vi "MH_WRabbitGetSFPData.vi"(8 "error in (no error)":errorcluster, 11 "devidx":i32) -> (0 "error out":errorcluster, 1 "dRxs":i32[](array[numeric]), 2 "dTxs":i32[](array[numeric]), 3 "return type":i32, 4 "alphas":i32[](array[numeric]), 5 "sfpnames":string[](array[string]))   [LabVIEW 2019]
uses:
  MH_DllPath_global.vi
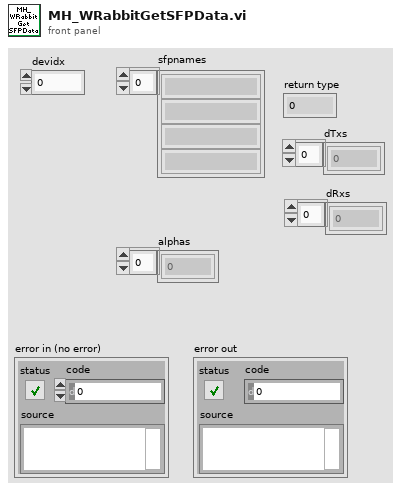
[diagram p1: front panel]
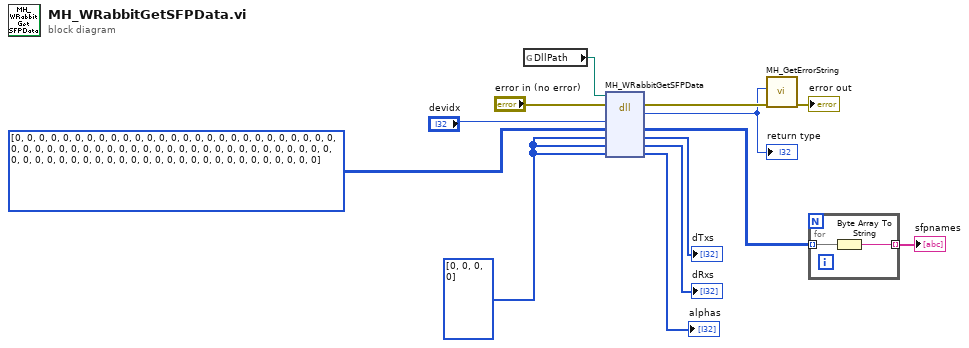
[diagram p0: block diagram]
diagram:
  w7 = i32[] [0, 0, 0, 0] ("dTxs")
  n1 = global read "MH_DllPath_global.vi" "DllPath"() -> (w11:path)
  n2 = dll-call lib="MHLib64.dll" fn="MH_WRabbitGetSFPData"(path in=w11, error in="error in (no error)", "devidx"="devidx", "sfpnames"=u8[][] [[0, 0, 0, 0, 0, 0, 0, 0, 0, 0, 0, 0, 0, 0, 0, 0, 0, 0, 0, 0], [0, 0, 0, 0, 0, 0, 0, 0, 0, 0, 0, 0, 0, 0, 0, 0, 0, 0, 0, 0], [0, 0, 0, 0, 0, 0, 0, 0, 0, 0, 0, 0, 0, 0, 0, 0, 0, 0, 0, 0], [0, 0, 0, 0, 0, 0, 0, 0, 0, 0, 0, 0, 0, 0, 0, 0, 0, 0, 0, 0]], "dTxs"=w7, "dRxs"=w7, "alphas"=w7) -> (error out=w10:errorcluster, "return type"=w9:i32, "sfpnames"=w2:u8[][], "dTxs"=→"dTxs":i32[], "dRxs"=→"dRxs":i32[], "alphas"=→"alphas":i32[])  [unwired: 2 in, 1 out]
  "return type" <- w9
  n3 = call "MH_GetErrorString.vi"("error in (no error)"=w10, "code"=w9) -> ("error out"=→"error out":errorcluster)  [unwired: 7 in, 2 out]
  n4 = for {
    tunnel: w2 -> [w15] mode=indexing
    tunnel: [w14] -> w1 mode=indexing
    n5 = Byte Array To String(unsigned byte array=w15) -> (string=w14:string)
  }
  "sfpnames" <- w1
